vi "Get Stop Values.vi"(8 "error in (no error)":errorcluster, 11 "Output Sequencer in":refnum<class "Output Sequencer.lvclass">) -> (0 "error out":errorcluster, 1 "Digital Values to Write":bool[](array[boolean]), 2 "Analog Values to Write":dbl[](array[numeric]), 3 "Output Sequencer out":refnum<class "Output Sequencer.lvclass">)   [LabVIEW 2020, in "Output Sequencer.lvlib" / "Output Sequencer.lvclass"]
uses:
  Output Sequencer.lvclass
  Output Sequencer.lvclass/Output Sequencer.ctl
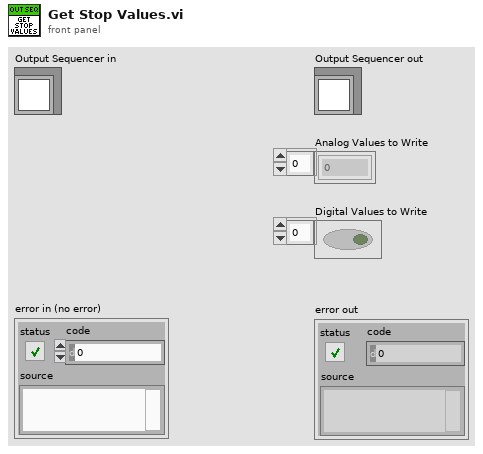
[diagram p1: front panel]
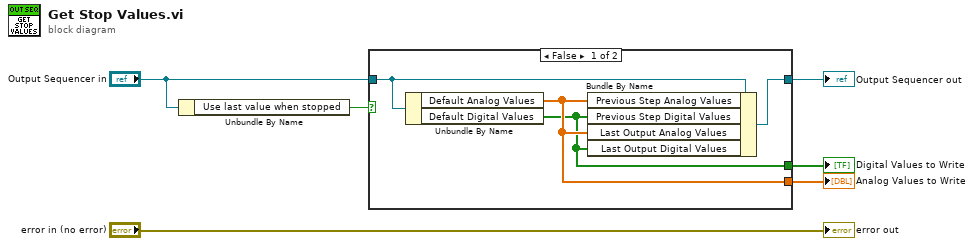
[diagram p0: block diagram]
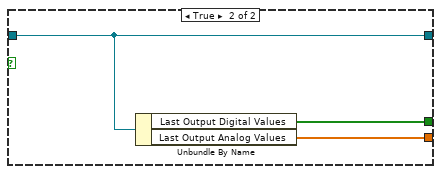
[diagram p2: hidden frame]
diagram:
  n1 = Unbundle By Name("Output Sequencer in") -> ("Use last value when stopped"=w2:bool)
  n2 = case shown="False" w2 {
    tunnel: "Output Sequencer in" -> [w10 w13]
    tunnel: [w9 w13] -> w4
    tunnel: [w8 w12] -> w5
    tunnel: [w7 w11] -> w6
    frame False {
      n3 = Unbundle By Name(w10) -> ("Default Analog Values"=w8:dbl[], "Default Digital Values"=w7:bool[])
      n4 = Bundle By Name(cluster=w10, "Previous Step Analog Values"=w8, "Previous Step Digital Values"=w7, "Last Output Analog Values"=w8, "Last Output Digital Values"=w7) -> (w9:refnum<class "Output Sequencer.lvclass">)
    }
    frame True {
      n5 = Unbundle By Name(w13) -> ("Last Output Digital Values"=w11:bool[], "Last Output Analog Values"=w12:dbl[])
    }
  }
  "Digital Values to Write" <- w6
  "Analog Values to Write" <- w5
  "Output Sequencer out" <- w4
  "error out" <- "error in (no error)"
